vi "zmq_setsocketopt.vi"(4 "error in":errorcluster, 5 "value":variant, 6 "option":T1=enum."ZMQ_SWAP", 7 "socket in":refnum<class "zmq_socket.lvclass">) -> (0 "error out":errorcluster, 3 "socket out":refnum<class "zmq_socket.lvclass">)   [LabVIEW 2019, in "zeromq.lvlib" / "zmq_socket.lvclass"]
doc: "Sets the specified <b>option</b> to the given <b>value</b>. The type of data connected to value must match that expected by the option (see the API documentation).\n\nNote that LabVIEW strings are used for \"raw\" data.\n\nDetailed API documentation: http://api.zeromq.org/3-2:zmq-setsockopt"
uses:
  zmq_socket.lvclass
  socket_options.ctl
  zmq_socket.lvclass/zmq_socket.ctl
  zeromq.lvlib
panel:
  out "option code":i32
  # "ØMQ"
  # "labview"
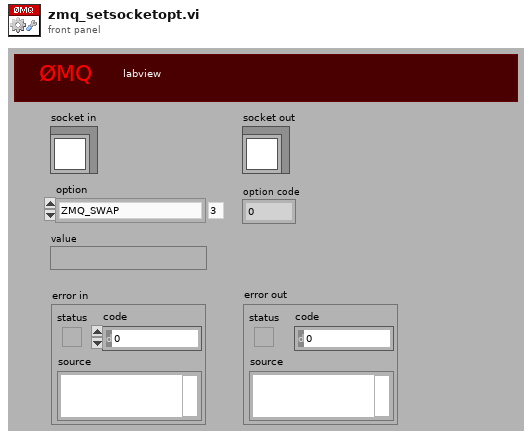
[diagram p1: front panel]
types:
  T1 = typedef "zeromq.lvlib/socket_options.ctl" = enum8{"NONE", "ZMQ_HWM", "<2>", "ZMQ_SWAP", "ZMQ_AFFINITY", "ZMQ_IDENTITY", "ZMQ_SUBSCRIBE", "ZMQ_UNSUBSCRIBE", "ZMQ_RATE", "ZMQ_RECOVERY_IVL", "ZMQ_MCAST_LOOP", "ZMQ_SNDBUF", "ZMQ_RCVBUF", "ZMQ_RCVMORE", "ZMQ_FD", "ZMQ_EVENTS", "ZMQ_TYPE", "ZMQ_LINGER", "ZMQ_RECONNECT_IVL", "ZMQ_BACKLOG", "ZMQ_RECOVERY_IVL_MSEC", "ZMQ_RECONNECT_IVL_MAX", "ZMQ_MAXMSGSIZE", "ZMQ_SNDHWM", "ZMQ_RCVHWM", "ZMQ_MULTICAST_HOPS", "<26>", "ZMQ_RCVTIMEO", "ZMQ_SNDTIMEO", "<29>", "<30>", "ZMQ_IPV4ONLY", "ZMQ_LAST_ENDPOINT", "ZMQ_ROUTER_MANDATORY", "ZMQ_TCP_KEEPALIVE", "ZMQ_TCP_KEEPALIVE_CNT", "ZMQ_TCP_KEEPALIVE_IDLE", "ZMQ_TCP_KEEPALIVE_INTVL", "ZMQ_TCP_ACCEPT_FILTER", "ZMQ_DELAY_ATTACH_ON_CONNECT", "ZMQ_XPUB_VERBOSE"}
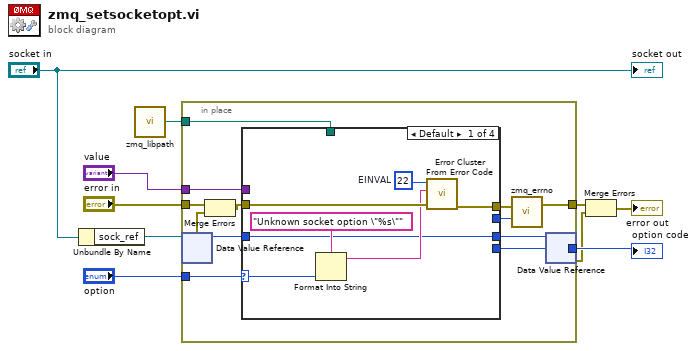
[diagram p0: block diagram]
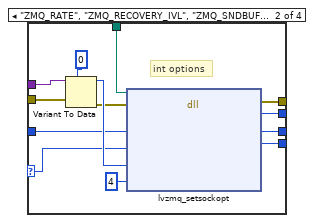
[diagram p2: hidden frame]
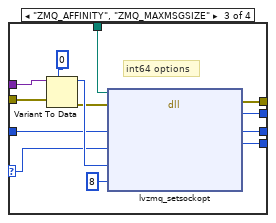
[diagram p3: hidden frame]
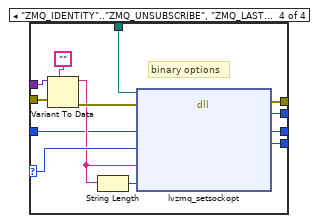
[diagram p4: hidden frame]
diagram:
  n1 = Unbundle By Name("socket in") -> ("sock_ref"=w4:refnum<data-value>)
  n2 = call "zmq_libpath.vi"() -> ("path"=w3:path)
  n3 = in-place {
    in-place-border: [w20] -> w10
    in-place-border: "value" -> [w19]
    in-place-border: "error in" -> [w18]
    in-place-border: "option" -> [w17]
    in-place-border: [w16] -> w6
    in-place-border: w3 -> [w13]
    n4 = in-place-dvr #1(w4) -> (w15:u64, w11:errorcluster)
    n5 = Merge Errors(w18, w11) -> (w12:errorcluster)
    n6 = case shown="Default" w17 {
      selector: w17 -> [w26 w35 w48 w62]
      tunnel: [w29 w42 w55 w68] -> w22
      tunnel: [_ w41 w54 w67] -> w21
      tunnel: w19 -> [_ w40 w53 w66]
      tunnel: w12 -> [w27 w37 w50 w64]
      tunnel: [_ w33 w46 w59] -> w16
      tunnel: w15 -> [w23 w32 w45 w57]
      tunnel: [w23 w31 w44 w58] -> w14
      tunnel: w13 -> [_ w30 w43 w56]
      frame Default {
        w28 = 22  # EINVAL
        n7 = Format Into String(format string="Unknown socket option \"%s\"", w26) -> (resulting string=w24:string)  [unwired: 2 in, 1 out]
        n8 = call <vilib>:"Error Cluster From Error Code.vi"("error in (no error)"=w27, "error message (\"\")"=w24, "error code (0)"=w28) -> ("error out"=w29:errorcluster)  [unwired: 6 in]
      }
      frame "ZMQ_RATE", "ZMQ_RECOVERY_IVL", "ZMQ_SNDBUF".."ZMQ_RECONNECT_IVL_MAX", "ZMQ_SNDHWM".."ZMQ_MULTICAST_HOPS", "ZMQ_RCVTIMEO", "ZMQ_SNDTIMEO", "ZMQ_IPV4ONLY", "ZMQ_ROUTER_MANDATORY".."ZMQ_XPUB_VERBOSE" {
        # "int options"
        n9 = Variant To Data(error in=w37, type=0, Variant=w40) -> (data=w39:i32, error out=w36:errorcluster)
        n10 = dll-call lib="?" fn="lvzmq_setsockopt"(path in=w30, error in=w36, "socket"=w32, "option"=w35, "data"=w39, "len"=u32 4) -> (error out=w42:errorcluster, "return type"=w41:i32, "socket"=w31:u64, "option"=w33:i32)  [unwired: 3 in, 1 out]
      }
      frame "ZMQ_AFFINITY", "ZMQ_MAXMSGSIZE" {
        # "int64 options"
        n11 = Variant To Data(error in=w50, type=i64 0, Variant=w53) -> (data=w52:i64, error out=w49:errorcluster)
        n12 = dll-call lib="?" fn="lvzmq_setsockopt"(path in=w43, error in=w49, "socket"=w45, "option"=w48, "data"=w52, "len"=u32 8) -> (error out=w55:errorcluster, "return type"=w54:i32, "socket"=w44:u64, "option"=w46:i32)  [unwired: 3 in, 1 out]
      }
      frame "ZMQ_IDENTITY".."ZMQ_UNSUBSCRIBE", "ZMQ_LAST_ENDPOINT" {
        # "binary options"
        n13 = Variant To Data(error in=w64, type="", Variant=w66) -> (data=w60:string, error out=w63:errorcluster)
        n14 = String Length(string=w60) -> (length=w61:i32)
        n15 = dll-call lib="?" fn="lvzmq_setsockopt"(path in=w56, error in=w63, "socket"=w57, "option"=w62, "data"=w60, "len"=w61) -> (error out=w68:errorcluster, "return type"=w67:i32, "socket"=w58:u64, "option"=w59:i32)  [unwired: 3 in, 1 out]
      }
    }
    n16 = call "zmq_errno.vi"("retval"=w21, "error in"=w22) -> ("error out"=w20:errorcluster)  [unwired: 1 out]
    n17 = in-place-dvr #1(w14) -> (w1:errorcluster)  [unwired: 1 out]
  }
  "option code" <- w6
  n18 = Merge Errors(w10, w1) -> (→"error out":errorcluster)
  "socket out" <- "socket in"
